vi "Run Task.vi"(8 "error in (no error)":errorcluster, 11 "DAQmxTask in":refnum<class "DAQmxTask.lvclass">) -> (0 "error out":errorcluster, 3 "DAQmxTask out":refnum<class "DAQmxTask.lvclass">)   [LabVIEW 2018, in "DAQmxTask.lvclass"]
uses:
  DAQmxTask.lvclass
  DAQmxTask.lvclass/DAQmxTask.ctl
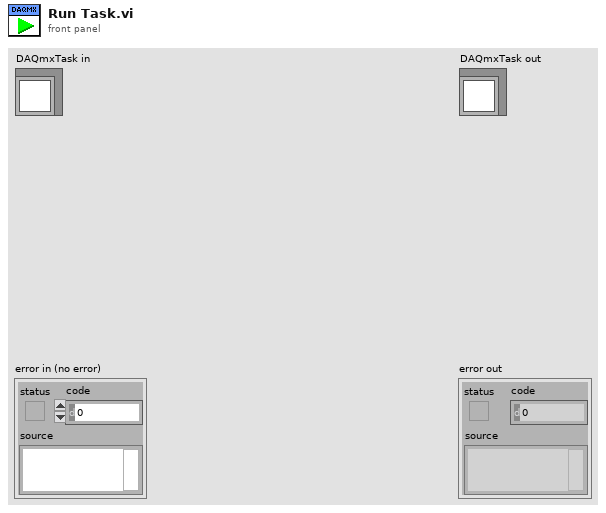
[diagram p1: front panel]
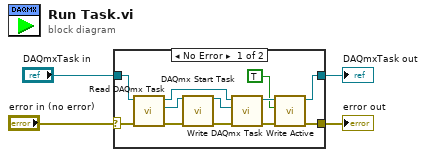
[diagram p0: block diagram]
diagram:
  n1 = case shown="No Error" "error in (no error)" {
    selector: "error in (no error)" -> [w15 w18]
    tunnel: [w8 w18] -> w3
    tunnel: [w6 w17] -> w1
    tunnel: "DAQmxTask in" -> [w16 w17]
    frame No Error {
      n2 = call "Read DAQmx Task.vi"("error in (no error)"=w15, "DAQmxTask in"=w16) -> ("error out"=w13:errorcluster, "DAQmx Task Name"=w14:refnum<k21>, "DAQmxTask out"=w10:refnum<class "DAQmxTask.lvclass">)  [unwired: 7 in]
      n3 = call <vilib>:"DAQmx Start Task.vi"("task/channels in"=w14, "error in"=w13) -> ("task out"=w11:refnum<k21>, "error out"=w12:errorcluster)  [unwired: 12 in]
      n4 = call "Write DAQmx Task.vi"("error in (no error)"=w12, "DAQmx Task Name"=w11, "DAQmxTask in"=w10) -> ("error out"=w9:errorcluster, "DAQmxTask out"=w7:refnum<class "DAQmxTask.lvclass">)  [unwired: 7 in]
      n5 = call-dynamic "Write Active.vi"("error in (no error)"=w9, "Active?"=TRUE, "DAQmxTask in"=w7) -> ("error out"=w8:errorcluster, "DAQmxTask out"=w6:refnum<class "DAQmxTask.lvclass">)  [unwired: 7 in]
    }
    frame Error {
    }
  }
  "error out" <- w3
  "DAQmxTask out" <- w1
